vi "yolov4_obj_detect.vi"(7 "Python session in":refnum<k35>, 8 "error in (no error)":errorcluster, 9 "Image Src":T1, 10 "Function name":string, 11 "Module path":path) -> (0 "BBoxes [y_min, x_min, y_max, x_max]":dbl[][](array[numeric]), 1 "Scores":dbl[](array[numeric]), 2 "Numbered classes":dbl[](array[numeric]), 3 "Number of detections":dbl, 4 "error out":errorcluster, 5 "Python session out":refnum<k35>)   [LabVIEW 2019]
uses:
  <vilib>/vision/Image Controls.llb/IMAQ Image.ctl
  0749c5da-743e-4ad5-b0f0-8c1a551efabe.vi
  <vilib>/Array/Sort 2D Array - Pop Stack.vi
  <vilib>/Array/Sort 2D Array - Push Stack.vi
  0749c5da-743e-4ad5-b0f0-8c1a551efabe.vi/e728fcae-d7e0-480a-bd69-4c5b20f56097.vi
  0749c5da-743e-4ad5-b0f0-8c1a551efabe.vi/a6fdb645-1efd-4d8c-828f-cf83d982203a.vi
  <vilib>/vision/NI_Vision_Development_Module.lvlib
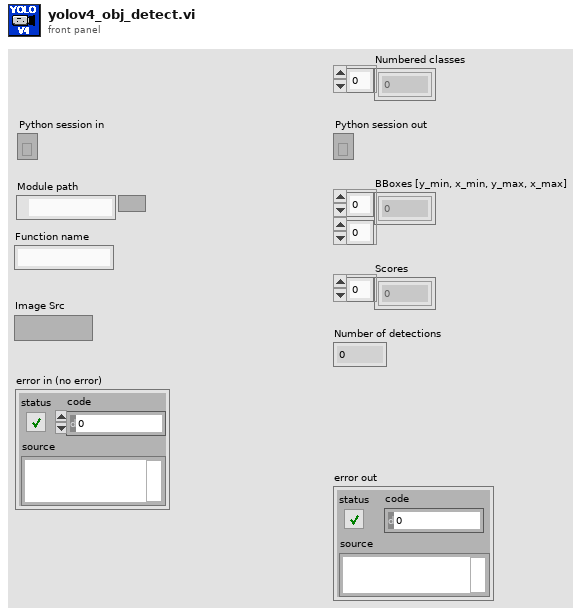
[diagram p1: front panel]
types:
  T1 = typedef "IMAQ Image.ctl" = refnum<image>
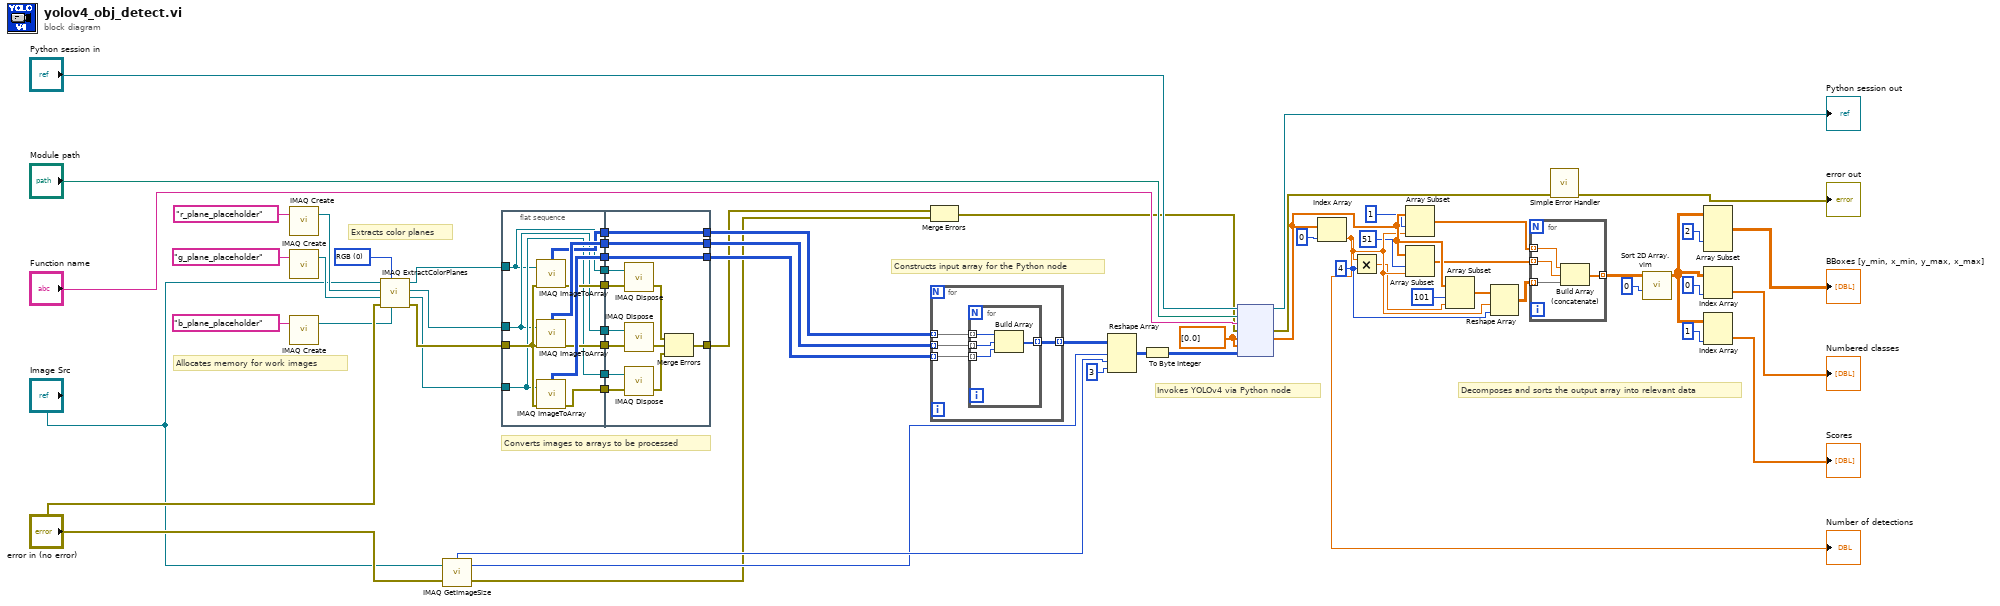
[diagram p0: block diagram]
diagram:
  w36 = u16 0 items=["RGB", "HSL", "HSV", "HSI"] ("Color Mode")
  w49 = dbl[] [0.0]
  w56 = 4 ("index (row)")
  # "Decomposes and sorts the output array into relevant data"
  # "Invokes YOLOv4 via Python node"
  # "Constructs input array for the Python node"
  # "Converts images to arrays to be processed"
  # "Extracts color planes"
  # "Allocates memory for work images"
  n1 = call "IMAQ Create"("Image Name"="r_plane_placeholder") -> ("New Image"=w29:T1)  [unwired: 4 in, 1 out]
  n2 = call "IMAQ Create"("Image Name"="g_plane_placeholder") -> ("New Image"=w27:T1)  [unwired: 4 in, 1 out]
  n3 = call "IMAQ Create"("Image Name"="b_plane_placeholder") -> ("New Image"=w25:T1)  [unwired: 4 in, 1 out]
  n4 = call "IMAQ ExtractColorPlanes"("Blue or Luma or Val or Inten Plane"=w25, "Color Mode"=w36, "error in (no error)"="error in (no error)", "Green or Sat Plane"=w27, "Red or Hue Plane"=w29, "Image Src"="Image Src") -> ("error out"=w18:errorcluster, "Blue or Luma or Val or Inten Plane out"=w12:T1, "Green or Sat Plane out"=w17:T1, "Red or Hue Plane out"=w16:T1)  [unwired: 2 in]
  n5 = call "IMAQ GetImageSize"("Image"="Image Src", "error in (no error)"="error in (no error)") -> ("Y Resolution"=w33:i32, "X Resolution"=w34:i32, "error out"=w2:errorcluster)  [unwired: 2 in]
  n6 = flat-sequence {
    tunnel: w18 -> [w72]
    tunnel: w12 -> [w65]
    tunnel: w17 -> [w64]
    tunnel: w16 -> [w63]
    tunnel: [w71] -> w11
    tunnel: [w70] -> w10
    tunnel: [w69] -> w9
    tunnel: [w68] -> w8
    tunnel: [w67] -> w7
    tunnel: [w66] -> w6
    tunnel: [w65] -> w5
    tunnel: [w64] -> w4
    tunnel: [w63] -> w3
    tunnel: [w85] -> w15
    tunnel: w11 -> [w85]
    tunnel: [w84] -> w14
    tunnel: w10 -> [w84]
    tunnel: [w83] -> w13
    tunnel: w9 -> [w83]
    tunnel: w8 -> [w82]
    tunnel: w7 -> [w81]
    tunnel: w6 -> [w80]
    tunnel: w5 -> [w76]
    tunnel: w4 -> [w75]
    tunnel: w3 -> [w74]
    tunnel: [w73] -> w1
    frame #0 {
      n7 = call "IMAQ ImageToArray"("error in (no error)"=w72, "Image"=w63) -> ("error out"=w68:errorcluster, "Image Pixels (U8)"=w69:u8[][])  [unwired: 2 in, 3 out]
      n8 = call "IMAQ ImageToArray"("error in (no error)"=w72, "Image"=w64) -> ("error out"=w67:errorcluster, "Image Pixels (U8)"=w70:u8[][])  [unwired: 2 in, 3 out]
      n9 = call "IMAQ ImageToArray"("error in (no error)"=w72, "Image"=w65) -> ("error out"=w66:errorcluster, "Image Pixels (U8)"=w71:u8[][])  [unwired: 2 in, 3 out]
    }
    frame #1 {
      n10 = call "IMAQ Dispose"("Image"=w74, "error in (no error)"=w82) -> ("error out"=w79:errorcluster)  [unwired: 4 in]
      n11 = call "IMAQ Dispose"("Image"=w75, "error in (no error)"=w81) -> ("error out"=w78:errorcluster)  [unwired: 4 in]
      n12 = call "IMAQ Dispose"("Image"=w76, "error in (no error)"=w80) -> ("error out"=w77:errorcluster)  [unwired: 4 in]
      n13 = Merge Errors(w79, w78, w77) -> (w73:errorcluster)
    }
  }
  n14 = Merge Errors(w1, w2) -> (w24:errorcluster)
  n15 = for {
    tunnel: w13 -> [w89] mode=indexing
    tunnel: w14 -> [w88] mode=indexing
    tunnel: w15 -> [w87] mode=indexing
    tunnel: [w86] -> w37 mode=indexing
    n16 = for {
      tunnel: w89 -> [w93] mode=indexing
      tunnel: w88 -> [w92] mode=indexing
      tunnel: w87 -> [w91] mode=indexing
      tunnel: [w90] -> w86 mode=indexing
      n17 = Build Array(w93, w92, w91) -> (w90:u8[])
    }
  }
  n18 = Reshape Array(w37, w33, w34, 3 ("dimension size")) -> (w38:u8[][][])
  n19 = To Byte Integer(number=w38) -> (8bit integer=w31:i8[][][])
  n20 = node("Python session in", "Module path", "Function name", w24, w49, w49, w31) -> (→"Python session out":refnum<k35>, w20:errorcluster, w62:dbl[])  [unwired: 2 in, 2 out]
  n21 = Index Array(array=w62, index=0) -> (element=w57:dbl)
  "Number of detections" <- w57
  n22 = Multiply(x=w57, y=w56) -> (x*y=w50:dbl)
  n23 = Array Subset(array=w62, index=1, length=w57) -> (w48:dbl[])
  n24 = Array Subset(array=w62, index=51, length=w57) -> (w47:dbl[])
  n25 = Array Subset(array=w62, index=101, length=w50) -> (w51:dbl[])
  n26 = Reshape Array(w51, w57, w56) -> (w46:dbl[][])
  n27 = for {
    tunnel: w48 -> [w97] mode=indexing
    tunnel: w47 -> [w96] mode=indexing
    tunnel: w46 -> [w95] mode=indexing
    tunnel: [w94] -> w45 mode=indexing
    n28 = Build Array (concatenate)(w97, w96, w95) -> (w94:dbl[])
  }
  n29 = call <vilib>:"Simple Error Handler.vi"("error in (no error)"=w20) -> ("error out"=→"error out":errorcluster)  [unwired: 4 in, 4 out]
  n30 = call "Sort 2D Array.vim"("index"=0, "2D array"=w45) -> ("sorted 2D array"=w41:dbl[][])  [unwired: 8 in, 1 out]
  n31 = Array Subset(array=w41, index (col)=2 ("index")) -> (→"BBoxes [y_min, x_min, y_max, x_max]":dbl[][])  [unwired: 3 in]
  n32 = Index Array(array=w41, index (col)=0 ("disabled index (col)")) -> (element=→"Numbered classes":dbl[])  [unwired: 1 in]
  n33 = Index Array(array=w41, index (col)=1 ("disabled index (col)")) -> (element=→"Scores":dbl[])  [unwired: 1 in]
